vi "Initialize Configure Initiate Scope with TClk.vi"(8 "error in (no error)":errorcluster, 10 "ref trigger source":string, 11 "scope info map":T3(c390)) -> (0 "error out":errorcluster, 3 "scope handles":refnum<k15>[](array[refnum]))   [LabVIEW 2021, in "PMIC Common.lvlib"]
uses:
  PMIC Common.lvlib
  <instrlib>/niScope/Configure/Trigger/niScope Configure Trigger Digital.vi
  <instrlib>/niScope/Controls/niScope vertical coupling.ctl
  Scope Parameters.ctl
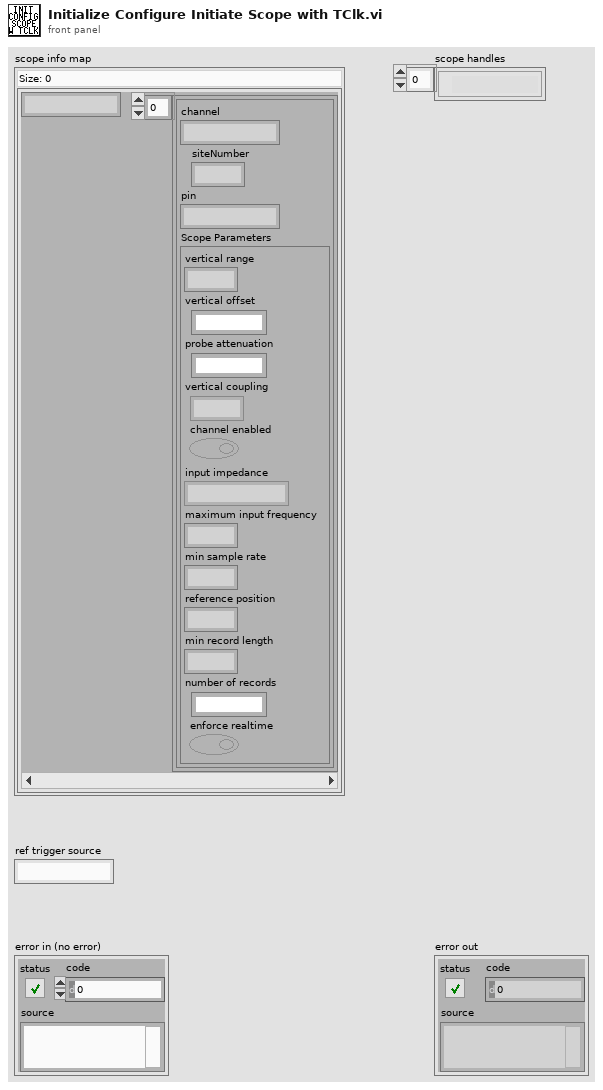
[diagram p1: front panel]
types:
  T1 = typedef "PMIC Common.lvlib/Scope Parameters.ctl" = cluster{"vertical range":dbl, "vertical offset":dbl, "probe attenuation":dbl, "vertical coupling":T2, "channel enabled":bool, "input impedance":u32, "maximum input frequency":dbl, "min sample rate":dbl, "reference position":dbl, "min record length":i32, "number of records":i32, "enforce realtime":bool}
  T2 = typedef "niScope vertical coupling.ctl" = i32
  T3 = map{string, cluster{"channel":string, "siteNumber":i32, "pin":string, "Scope Parameters":T1}[]}
  T4 = cluster{"channel":string, "siteNumber":i32, "pin":string, "Scope Parameters":T1}[]
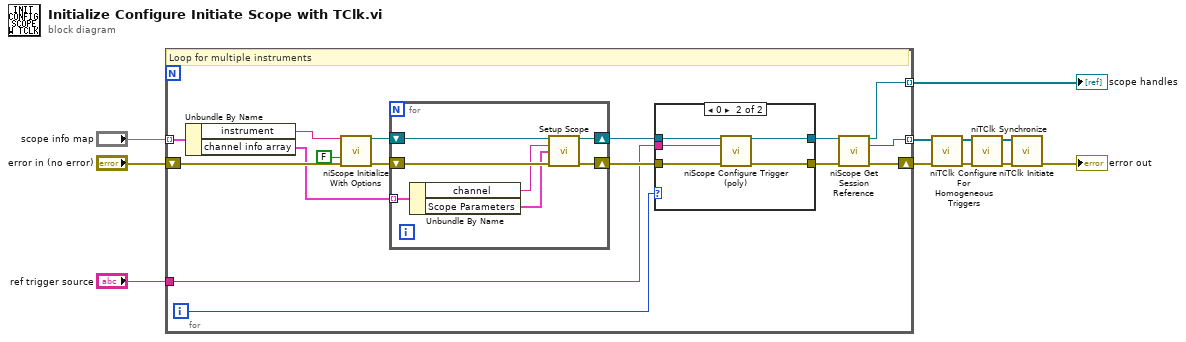
[diagram p0: block diagram]
diagram:
  n1 = for {
    tunnel: "ref trigger source" -> [w21]
    shift-right: [w17] -> w5
    shift-left: "error in (no error)" -> [w27]
    tunnel: [w16] -> w9 mode=indexing
    tunnel: "scope info map" -> [w15] mode=indexing
    tunnel: [w12] -> w10 mode=indexing
    i -> [w20]
    # "Loop for multiple instruments"
    n2 = Unbundle By Name(w15) -> ("instrument"=w14:string, "channel info array"=w13:T4)
    n3 = call <instrlib>:"niScope Initialize With Options.vi"("resource name"=w14, "reset device"=FALSE, "error in"=w27) -> ("instrument handle"=w24:refnum<k15>, "error out"=w25:errorcluster)  [unwired: 11 in]
    n4 = for {
      shift-right: [w31] -> w22
      shift-left: w25 -> [w34]
      shift-right: [w32] -> w23
      shift-left: w24 -> [w33]
      tunnel: w13 -> [w28] mode=indexing
      n5 = Unbundle By Name(w28) -> ("channel"=w30:string, "Scope Parameters"=w29:T1)
      n6 = call "Setup Scope.vi"("instrument handle"=w33, "channels"=w30, "Scope Parameters"=w29, "error in"=w34) -> ("instrument handle out"=w32:refnum<k15>, "error out"=w31:errorcluster)  [unwired: 10 in]
    }
    n7 = case shown="0" w20 {
      tunnel: w23 -> [w35 w41]
      tunnel: w22 -> [w36 w40]
      tunnel: w21 -> [_ w39]
      tunnel: [w36 w37] -> w18
      tunnel: [w35 w38] -> w19
      frame Default {
      }
      frame 0 {
        n8 = call-poly <instrlib>:"niScope Configure Trigger (poly).vi"("instrument handle"=w41, "trigger source"=w39, "error in"=w40) -> ("instrument handle out"=w38:refnum<k15>, "error out"=w37:errorcluster)  [unwired: 11 in]
      }
    }
    n9 = call <instrlib>:"niScope Get Session Reference.vi"("instrument handle"=w19, "error in"=w18) -> ("instrument handle out"=w12:refnum<k15>, "session reference"=w16:refnum<k20>, "error out"=w17:errorcluster)  [unwired: 11 in]
  }
  "scope handles" <- w10
  n10 = call <instrlib>:"niTClk Configure For Homogeneous Triggers.vi"("error in (no error)"=w5, "sessions"=w9) -> ("error out"=w6:errorcluster, "sessions out"=w4:refnum<k20>[])  [unwired: 8 in]
  n11 = call <instrlib>:"niTClk Synchronize.vi"("error in (no error)"=w6, "sessions"=w4) -> ("error out"=w7:errorcluster, "sessions out"=w3:refnum<k20>[])  [unwired: 8 in]
  n12 = call <instrlib>:"niTClk Initiate.vi"("error in (no error)"=w7, "sessions"=w3) -> ("error out"=→"error out":errorcluster)  [unwired: 8 in, 1 out]
